vi "Initialize.vi"(8 "error in (no error)":errorcluster, 10 "PlayerMoves":T1[](array[typedef]), 11 "PlayerName":string) -> (0 "error out":errorcluster)   [LabVIEW 2015, in "ReplayBot.lvlib"]
uses:
  ReplayBot.lvlib
  TronVIEWBotAPI/MovementDirection.ctl
  TronVIEWBotAPI/TronVIEWBotAPI.lvlib
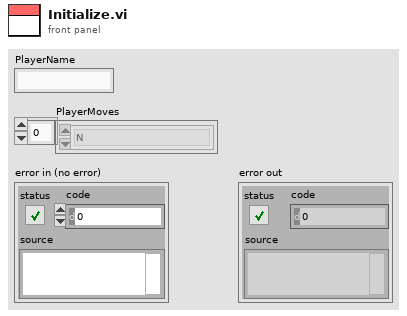
[diagram p1: front panel]
types:
  T1 = typedef "TronVIEWBotAPI.lvlib/MovementDirection.ctl" = enum16{"N", "S", "W", "E"}
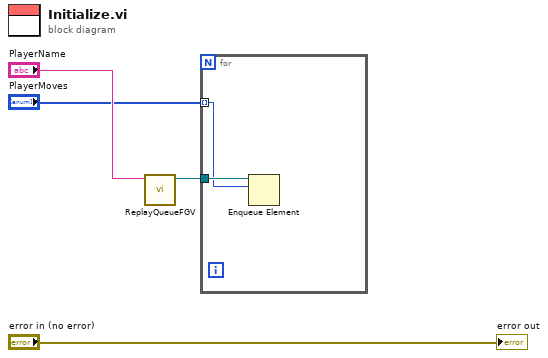
[diagram p0: block diagram]
diagram:
  n1 = call "ReplayQueueFGV.vi"("PlayerName"="PlayerName") -> ("queue out"=w3:refnum<queue>)  [unwired: 10 in]
  n2 = for {
    tunnel: w3 -> [w6]
    tunnel: "PlayerMoves" -> [w5] mode=indexing
    n3 = Enqueue Element(queue=w6, element=w5) -> ()  [unwired: 2 in, 3 out]
  }
  "error out" <- "error in (no error)"
